vi "json_test_read.vi"(8 "error in":errorcluster, 11 "Parent VI Path":path) -> (0 "error out":errorcluster, 3 "value":T1)   [LabVIEW 2020]
panel:
  in  "text":string
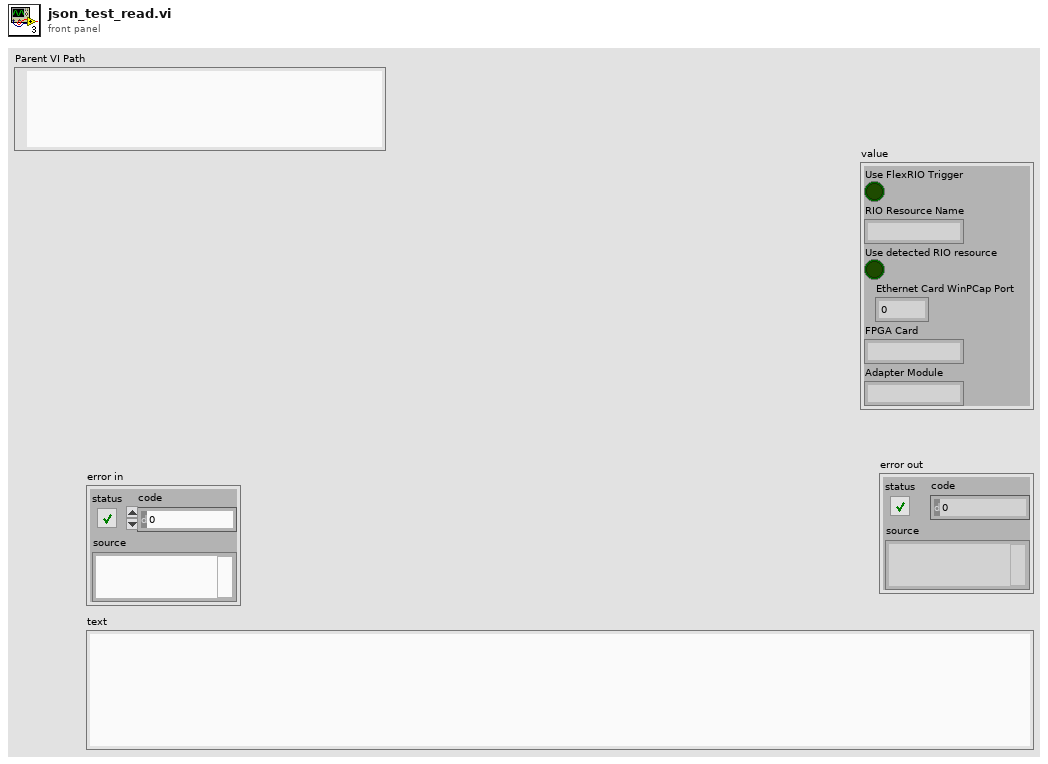
[diagram p1: front panel]
types:
  T1 = cluster{"Use FlexRIO Trigger":bool, "RIO Resource Name":string, "Use detected RIO resource":bool, "Ethernet Card WinPCap Port ":i16, "FPGA Card":string, "Adapter Module":string}
  T2 = enum32{"invalid app kind", "Development System", "Run Time System", "Student Edition", "Embedded LabVIEW", "Evaluation", "Custom"}
  T3 = enum16{"open", "replace", "create", "open or create", "replace or create", "replace or create with confirmation"}
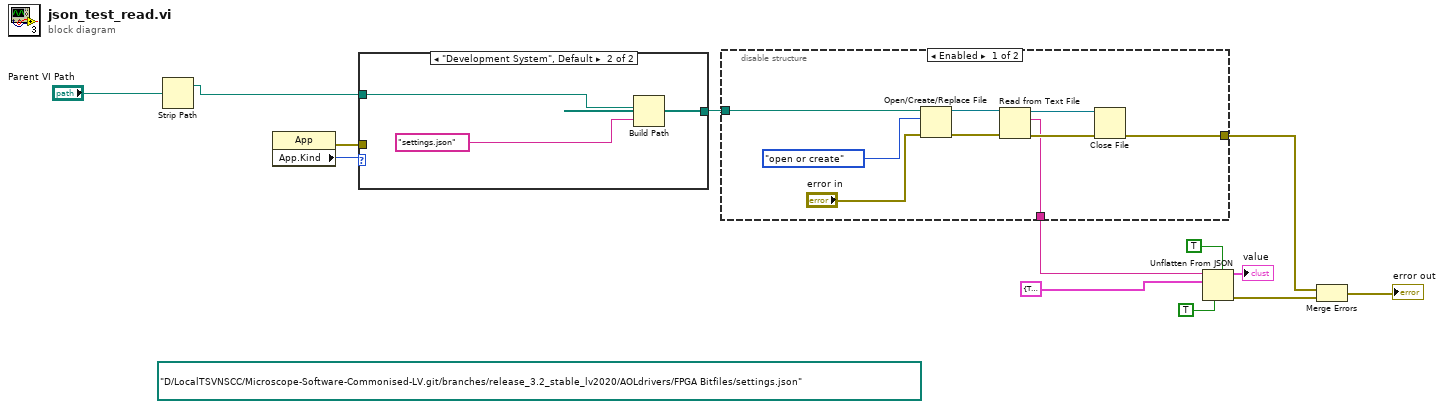
[diagram p0: block diagram]
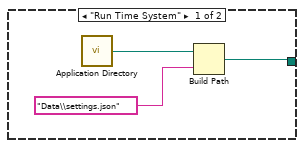
[diagram p2: hidden frame]
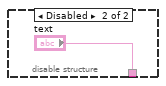
[diagram p3: hidden frame]
diagram:
  (unwired) path "D:/LocalTSVNSCC/Microscope-Software-Commonised-LV.git/branches/release_3.2_stable_lv2020/AOLdrivers/FPGA Bitfiles/settings.json" ("file path (use dialog)")
  n1 = Strip Path(path="Parent VI Path") -> (stripped path=w1:path)  [unwired: 1 out]
  n2 = property class="App"() -> (error out=w3:errorcluster, "App.Kind"=w4:T2)  [unwired: 2 in, 1 out]
  n3 = case shown="\"Development System\", Default" w4 {
    tunnel: [w14 w18] -> w5
    tunnel: w3 -> [_ _]
    tunnel: w1 -> [_ w17]
    frame "Run Time System" {
      n4 = call <vilib>:"Application Directory.vi"() -> ("Application Directory"=w16:path)
      n5 = Build Path(base path=w16, name or relative path="Data\\settings.json") -> (appended path=w14:path)
    }
    frame "Development System", Default {
      n6 = Build Path(base path=w17, name or relative path="settings.json") -> (appended path=w18:path)
    }
  }
  n7 = disable-structure shown="Enabled" {
    disable-tunnel: [w23 "text"] -> w13
    disable-tunnel: [w21 _] -> w8
    disable-tunnel: w5 -> [w20 _]
    frame Enabled {
      n8 = Open/Create/Replace File(file path (use dialog)=w20, error in="error in", operation (0:open)=T3."open or create") -> (refnum out=w27:refnum<file>, error out=w28:errorcluster)  [unwired: 3 in, 1 out]
      n9 = Read from Text File(file (use dialog)=w27, error in=w28) -> (refnum out=w25:refnum<file>, text=w23:string, error out=w26:errorcluster)  [unwired: 2 in, 1 out]
      n10 = Close File(refnum=w25, error in=w26) -> (error out=w21:errorcluster)  [unwired: 1 out]
    }
    frame Disabled {
    }
  }
  n11 = Unflatten From JSON(enable LabVIEW extensions? (T)=TRUE, JSON string=w13, type and defaults=T1 {"Use FlexRIO Trigger"=TRUE, "RIO Resource Name"="", "Use detected RIO resource"=FALSE, "Ethernet Card WinPCap Port "=0, "FPGA Card"="", "Adapter Module"=""} ("Controls 2"), default null elements? (F)=TRUE) -> (value=→"value":T1, error out=w7:errorcluster)  [unwired: 3 in]
  n12 = Merge Errors(w8, w7) -> (→"error out":errorcluster)
